vi "First result.vi"(8 "entrée d'erreur (pas d'erreur)":errorcluster, 11 "Zigbee_Send_Msg en entrée":refnum<class "Zigbee_Send_Msg.lvclass">) -> (0 "sortie d'erreur":errorcluster, 2 "Chaîne OUT":string, 3 "Zigbee_Send_Msg en sortie":refnum<class "Zigbee_Send_Msg.lvclass">)   [LabVIEW 2020, in "Library Test.lvlib" / "Zigbee_Send_Msg.lvclass"]
uses:
  Zigbee_Send_Msg.lvclass
  C:/Users/ngarcin/OneDrive - Altyor/Standard TB/Suite TB45/Class/Test/Test (Default)/Test (Default).lvclass
  Commun VI/TypeDef/Variable Printable.ctl
  Commun VI/Library Commun.lvlib
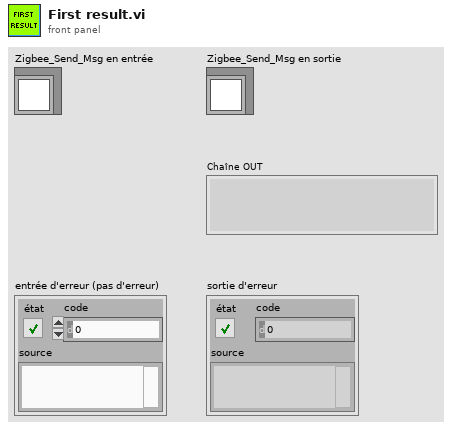
[diagram p1: front panel]
types:
  T1 = typedef "Variable Printable.ctl" = string
  T2 = enum16{"Get Variable", "Get All Variables", "Set Variable", "Delete Variable", "Delete All Variable"}
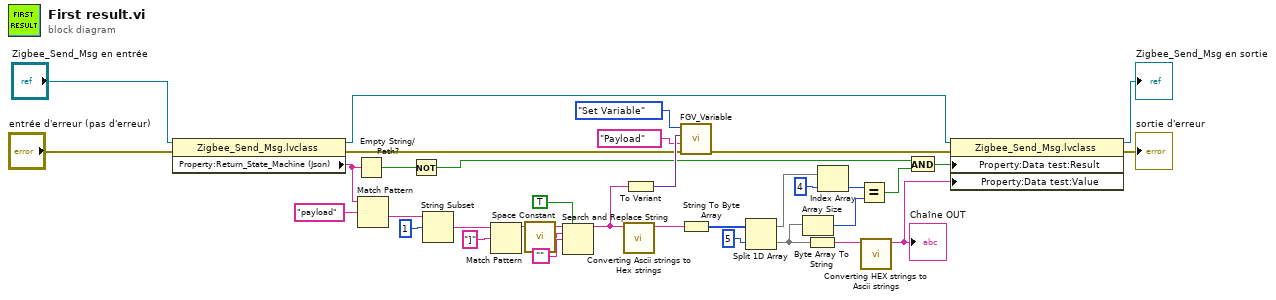
[diagram p0: block diagram]
diagram:
  n1 = property class="Zigbee_Send_Msg.lvclass"(reference="Zigbee_Send_Msg en entrée", error in="entrée d'erreur (pas d'erreur)") -> (reference out=w2:refnum<class "Zigbee_Send_Msg.lvclass">, error out=w31:errorcluster, "Property:Return_State_Machine (Json)"=w1:string)
  n2 = Empty String/Path?(string/path=w1) -> (empty?=w3:bool)
  n3 = Match Pattern(string=w1, regular expression="payload" ("expression régulière")) -> (after substring=w12:string)  [unwired: 1 in, 3 out]
  n4 = Not(x=w3) -> (.not. x?=w17:bool)
  n5 = String Subset(string=w12, offset (0)=1) -> (substring=w11:string)  [unwired: 1 in]
  n6 = Match Pattern(string=w11, regular expression="]" ("expression régulière")) -> (before substring=w34:string)  [unwired: 1 in, 3 out]
  n7 = call <vilib>:"Space Constant.vi"() -> ("String"=w14:string)
  n8 = Search and Replace String(replace all?=TRUE ("tout remplacer ? (F)"), input string=w34, search string=w14, replace string="") -> (result string=w35:string)  [unwired: 4 in, 3 out]
  n9 = call "Converting Ascii strings to Hex strings.vi"("result string"=w35) -> ("Chaîne"=w25:string)  [unwired: 10 in]
  n10 = To Variant(anything=w35) -> (Variant=w33:variant)
  n11 = call "FGV_Variable.vi"("error in (no error)"=w31, "Variable"=T1 "Payload" ("Variable Printable"), "Data In"=w33, "Function"=T2."Set Variable") -> ("error out"=w32:errorcluster)  [unwired: 5 in, 2 out]
  n12 = String To Byte Array(string=w25) -> (unsigned byte array=w18:u8[])
  n13 = Split 1D Array(array=w18, index=5 ("indice")) -> (first subarray=w20:u8[], second subarray=w24:u8[])
  n14 = Array Size(array=w24) -> (size(s)=w23:i32)
  n15 = Byte Array To String(unsigned byte array=w24) -> (string=w26:string)
  n16 = Index Array(array=w20, index=4 ("indice")) -> (element=w22:u8)
  n17 = Equal?(x=w22, y=w23) -> (x = y?=w27:bool)
  n18 = call "Converting HEX strings to Ascii strings.vi"("chaîne IN"=w26) -> ("Chaîne OUT"=w28:string)  [unwired: 9 in, 1 out]
  "Chaîne OUT" <- w28
  n19 = And(x=w17, y=w27) -> (x .and. y?=w16:bool)
  n20 = property class="Zigbee_Send_Msg.lvclass"(reference=w2, error in=w32, "Property:Data test:Result"=w16, "Property:Data test:Value"=w28) -> (reference out=→"Zigbee_Send_Msg en sortie":refnum<class "Zigbee_Send_Msg.lvclass">, error out=→"sortie d'erreur":errorcluster)
